vi "Create Digital Output.vi"(8 "error in (no error)":errorcluster, 10 "Params":variant, 11 "NI Digital Output in":refnum<class "NI Digital Output.lvclass">) -> (0 "error out":errorcluster, 3 "NI Digital Output out":refnum<class "NI Digital Output.lvclass">)   [LabVIEW 2020, in "NI DAQmx.lvlib" / "NI Digital Output.lvclass"]
uses:
  NI Digital Output.lvclass
  D:/WSGitHub/RTFWK/Realization/NI DAQmx Base/NI DAQmx Base.lvclass
  <vilib>/DAQmx/create/channels.llb/DAQmx Create Channel (DO-Digital Output).vi
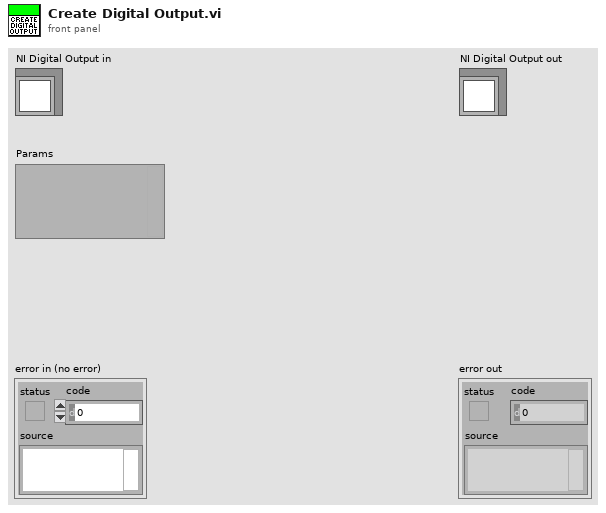
[diagram p1: front panel]
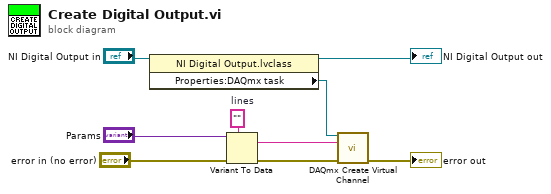
[diagram p0: block diagram]
diagram:
  w8 = ""  # lines
  n1 = property class="NI Digital Output.lvclass"(reference="NI Digital Output in") -> (reference out=→"NI Digital Output out":refnum<class "NI Digital Output.lvclass">, "Properties:DAQmx task"=w9:refnum<k21>)  [unwired: 1 in, 1 out]
  n2 = Variant To Data(error in="error in (no error)", type=w8, Variant="Params") -> (data=w6:string, error out=w7:errorcluster)
  n3 = call-poly <vilib>:"DAQmx Create Virtual Channel.vi"("task in"=w9, "lines"=w6, "error in"=w7) -> ("error out"=→"error out":errorcluster)  [unwired: 11 in, 1 out]
